vi "Feed Module Tags.vi"(0 "Feed Module Configs":T1[](array[typedef]) {"Settings"."Bronkhorst M14 Settings"."Smoothing Steps" min=1 step=1; "Settings"."Ismatech 3 Channel Settings"."Channel Number" min=0 max=3; "Settings"."Ismatech 3 Channel Settings"."Pump Number" min=1; "Settings"."PID range"."PID Low" min=0.0 max=100.0 format="%.2f"; "Settings"."PID range"."PID High" format="%.2f"; "Settings"."PID 2 Parameters"."PID gains"."derivative time (Td, min)" format="%.3f"; "Settings"."PID 2 Parameters"."PID gains"."integral time (Ti, min)" format="%.3f"; "Settings"."PID 2 Parameters"."PID gains"."proportional gain (Kc)" format="%.3f"; "Settings"."Bronkhorst M13 Flow Meter"."Smoothing Steps" min=1 step=1; "Settings"."ASIA Pump C"."channel" min=0 max=1 step=1; "Settings"."Ismatech"."Pump Number" min=1.0 max=20.0 step=1.0; "Settings"."Masterflex"."Pump Number" min=1.0 max=20.0 step=1.0}) -> (2 "All  Flow Meter Tags":string[](array[string]), 3 "All  Scale Tags":string[](array[string]), 4 "All  Numeric Tags":string[](array[string]), 6 "Pump Flow Tag":string, 8 "Feed Module Tag Names":T22, 10 "Feed Module Tags Array":T22[](array[typedef]), 12 "Scale Tag":string, 13 "All Boolean Tags":string[](array[string]), 14 "PID 2 Out Tag":string)   [LabVIEW 2018]
uses:
  Feed Module/Controls/Feed Module Tag Names Cluster.ctl
  Feed Module/Controls/Feed Module Config Cluster.ctl
  <vilib>/Utility/miscctls.llb/LVPoint32TypeDef.ctl
  Feed Module/Controls/Feed Module Settings Cluster.ctl
  Ismatec ISM 831C/Controls/Ismatech ISM831C Settings Cluster.ctl
  Masterflex 7550-30/Controls/Settings Cluster.ctl
  Mettler Toledo/Controls/Settings Cluster.ctl
  Bronkhorst M13 Flow Meter/Settings Cluster.ctl
  Measure Instrument/PID 2 Parameters Cluster.ctl
  Measure Instrument/PID Input Enum.ctl
  Measure Instrument/PID 2 Output Enum.ctl
  Tacmina QI/Tacmina QI DAQ Setting.ctl
  KNF Pump/Settings Cluster plus SIMDOS.ctl
  ASIA Pump/Pump Settings.ctl
  VICI M50 Party Mode/Settings Cluster.ctl
  FLOM Pump/Settings Cluster.ctl
  SSI PR Class/SSI PR or LD Settings Cluster.ctl
  Masterflex 75211/Masterflex 75211 DAQ Setting.ctl
  SSI PR Class/SSI P40 Settings Cluster.ctl
  Ismatec 78001/Ismatec 4083.ctl
  Bronkhorst M14 Flow Meter/Settings Cluster.ctl
  Tag VIs/Numeric Alarm Settings Cluster.ctl
  Feed Module/Feed Module.lvlib
  Masterflex 7550-30/Masterflex 7550-30.lvlib
  Ismatec ISM 831C/Ismatec ISM 831C.lvlib
  Tacmina QI/Tacmina QI.lvlib
  KNF Pump/KNF SIMDOS.lvlib
  VICI M50 Party Mode/VICI M6 M50 Party Mode.lvlib
  FLOM Pump/FLOM Pump.lvlib
  ASIA Pump.lvlib
  Mettler Toledo/Mettler Toledo.lvlib
  Bronkhorst M13 Flow Meter/Bronkhorst M13 Flow Meter.lvlib
  SSI PR Class/SSI PR or LD Pump.lvlib
  Masterflex 75211/Masterflex 75211.lvlib
  SSI PR Class/SSI P40 Pump.lvlib
  Ismatec 78001/Ismatec 4308.lvlib
  Bronkhorst M14 Flow Meter/Bronkhorst M14 Flow Meter.lvlib
panel:
  # "Output Instruments"
  # "Input Instruments"
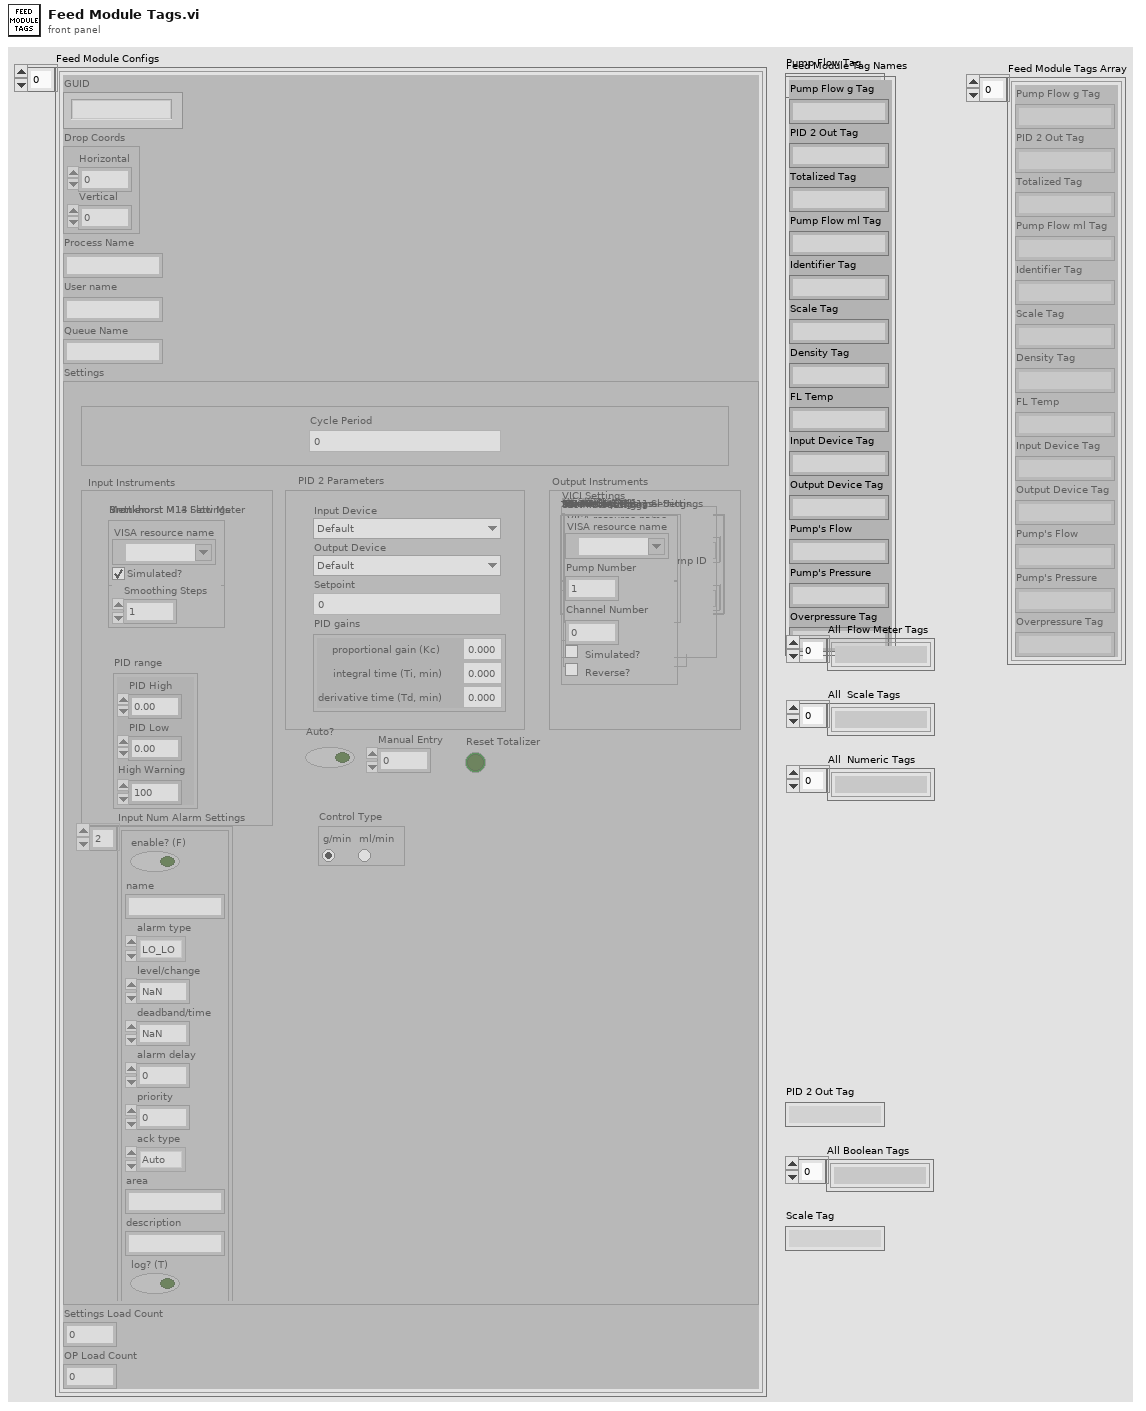
[diagram p1: front panel]
types:
  T1 = typedef "Feed Module.lvlib/Feed Module Config Cluster.ctl" = cluster{"GUID":string, "Drop Coords":T2, "Process Name":string, "User name":string, "Queue Name":string, "Settings":T3, "Settings Load Count":i32, "OP Load Count":i32}
  T2 = typedef "LVPoint32TypeDef.ctl" = cluster{"Horizontal":i32, "Vertical":i32}
  T3 = typedef "Feed Module.lvlib/Feed Module Settings Cluster.ctl" = cluster{"Cycle Period":dbl, "Ismatech":T4, "Masterflex":T5, "Mettler":T6, "Bronkhorst M13 Flow Meter":T7, "PID 2 Parameters":T8, "Manual Entry":dbl, "Auto?":bool, "PID range":cluster{"PID High":dbl, "PID Low":dbl, "High Warning":dbl}, "Tacmina Settings":T11, "KNF SIMDOS Settings":T12, "ASIA Pump C":T13, "VICI Settings":T14, "FLOM Settings":T15, "SSI PR/LD Settings":T16, "Masterflex 75211 Settings":T17, "SSI P40 Settings":T18, "Ismatech 3 Channel Settings":T19, "Bronkhorst M14 Settings":T20, "Reset Totalizer":bool, "Input Num Alarm Settings":T21[], "Control Type":enum32{"g/min", "ml/min"}}
  T4 = typedef "Ismatec ISM 831C.lvlib/Ismatech ISM831C Settings Cluster.ctl" = cluster{"VISA resource name":refnum<visa-resource-name>, "Simulated?":bool, "Pump Number":dbl, "Reverse?":bool}
  T5 = typedef "Masterflex 7550-30.lvlib/Settings Cluster.ctl" = cluster{"VISA resource name":refnum<visa-resource-name>, "Simulated?":bool, "Pump Number":dbl, "Reverse?":bool}
  T6 = typedef "Mettler Toledo.lvlib/Settings Cluster.ctl" = cluster{"VISA resource name":refnum<visa-resource-name>, "Simulated?":bool}
  T7 = typedef "Bronkhorst M13 Flow Meter.lvlib/Settings Cluster.ctl" = cluster{"VISA resource name":refnum<visa-resource-name>, "Simulated?":bool, "Smoothing Steps":i32}
  T8 = typedef "PID 2 Parameters Cluster.ctl" = cluster{"Input Device":T9, "Output Device":T10, "Setpoint":dbl, "PID gains":cluster{"proportional gain (Kc)":dbl, "integral time (Ti, min)":dbl, "derivative time (Td, min)":dbl}}
  T9 = typedef "PID Input Enum.ctl" = enum16{"Default", "Bronkhorst M13", "Bronkhorst M14", "Scale Rate of Change"}
  T10 = typedef "PID 2 Output Enum.ctl" = enum16{"Default", "Ismatec ISM 4308", "Ismatec ISM 831C", "Masterflex 7550-30", "VICI M6", "VICI M50", "Tacmina QI", "KNF SIMDOS", "ASIA Type C", "FLOM UI-22-11", "SSI PR/LD", "SSI P40", "Masterflex 75211-70"}
  T11 = typedef "Tacmina QI.lvlib/Tacmina QI DAQ Setting.ctl" = cluster{"Analog DAQ Task":refnum<k21>, "Digital DAQ Task":refnum<k21>}
  T12 = typedef "KNF SIMDOS.lvlib/Settings Cluster plus SIMDOS.ctl" = cluster{"VISA resource name":refnum<visa-resource-name>, "Simulated?":bool}
  T13 = typedef "ASIA Pump.lvlib/Pump Settings.ctl" = cluster{"ASIA Pump #":i32, "channel":i32, "Simulated":bool}
  T14 = typedef "VICI M6 M50 Party Mode.lvlib/Settings Cluster.ctl" = cluster{"VISA resource name":refnum<visa-resource-name>, "Pump ID":string, "Pump Head Vol":dbl, "Reverse?":bool, "Simulated?":bool}
  T15 = typedef "FLOM Pump.lvlib/Settings Cluster.ctl" = cluster{"VISA resource name":refnum<visa-resource-name>, "Simulated?":bool, "Pump Number":dbl}
  T16 = typedef "SSI PR or LD Pump.lvlib/SSI PR or LD Settings Cluster.ctl" = cluster{"VISA resource name":refnum<visa-resource-name>, "Simulated?":bool}
  T17 = typedef "Masterflex 75211.lvlib/Masterflex 75211 DAQ Setting.ctl" = cluster{"Analog DAQ Task":refnum<k21>, "Digital DAQ Task":refnum<k21>}
  T18 = typedef "SSI P40 Pump.lvlib/SSI P40 Settings Cluster.ctl" = cluster{"VISA resource name":refnum<visa-resource-name>, "Simulated?":bool}
  T19 = typedef "Ismatec 4308.lvlib/Ismatec 4083.ctl" = cluster{"VISA resource name":refnum<visa-resource-name>, "Pump Number":i16, "Channel Number":i16, "Simulated?":bool, "Reverse?":bool}
  T20 = typedef "Bronkhorst M14 Flow Meter.lvlib/Settings Cluster.ctl" = cluster{"VISA resource name":refnum<visa-resource-name>, "Simulated?":bool, "Smoothing Steps":i32}
  T21 = typedef "Numeric Alarm Settings Cluster.ctl" = cluster{"enable? (F)":bool, "name":string, "alarm type":enum16{"HI_HI", "HI", "LO", "LO_LO"}, "level/change":dbl, "deadband/time":dbl, "alarm delay":dbl, "priority":u32, "ack type":enum16{"Auto", "User", "None", "Each Occurrence"}, "area":string, "description":string, "log? (T)":bool}
  T22 = typedef "Feed Module.lvlib/Feed Module Tag Names Cluster.ctl" = cluster{"Pump Flow g Tag":string, "PID 2 Out Tag":string, "Totalized Tag":string, "Pump Flow ml Tag":string, "Identifier Tag":string, "Scale Tag":string, "Density Tag":string, "FL Temp":string, "Input Device Tag":string, "Output Device Tag":string, "Pump's Flow":string, "Pump's Pressure":string, "Overpressure Tag":string}
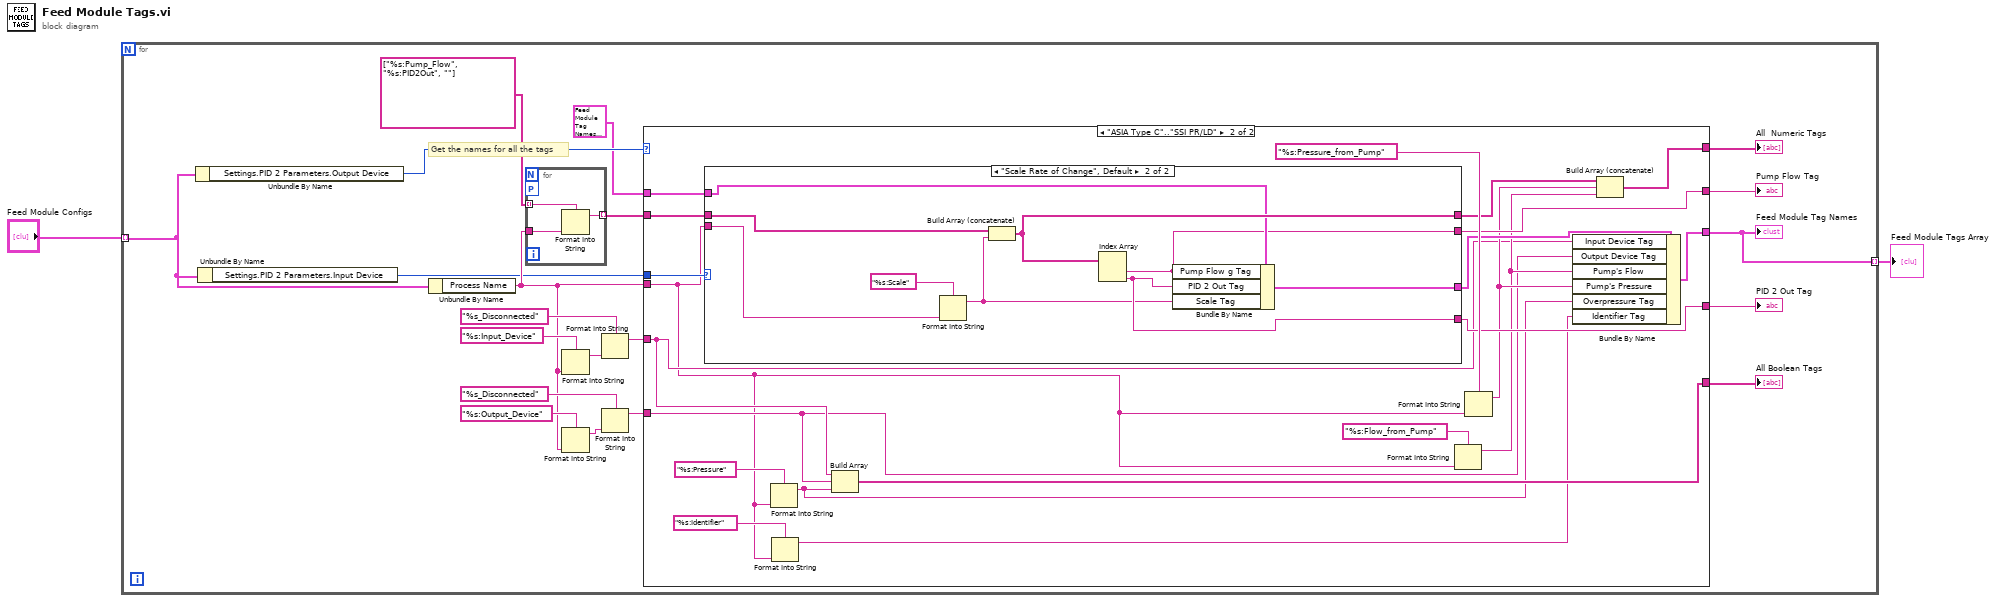
[diagram p0: block diagram]
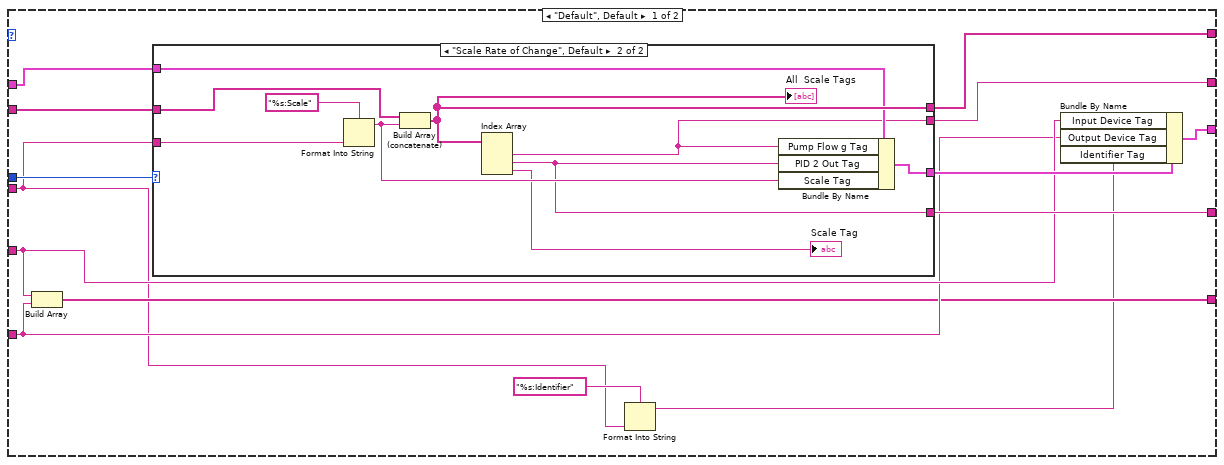
[diagram p2: hidden frame]
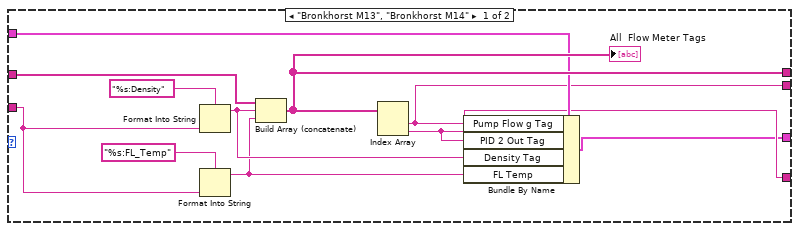
[diagram p3: hidden frame]
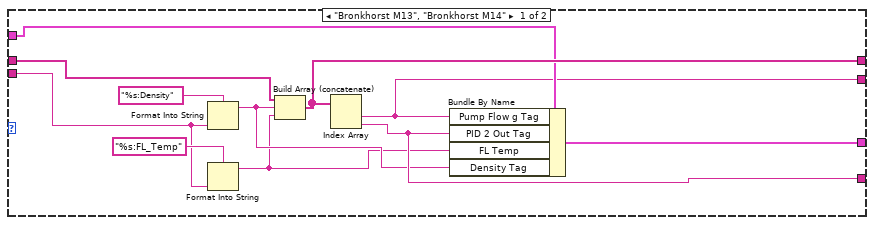
[diagram p4: hidden frame]
diagram:
  n1 = for {
    tunnel: "Feed Module Configs" -> [w5] mode=indexing
    tunnel: [w4] -> w2 mode=indexing
    # "Get the names for all the tags"
    n2 = Unbundle By Name(w5) -> ("Settings.PID 2 Parameters.Output Device"=w15:T10)
    n3 = Unbundle By Name(w5) -> ("Settings.PID 2 Parameters.Input Device"=w13:T9)
    n4 = Unbundle By Name(w5) -> ("Process Name"=w14:string)
    n5 = for {
      tunnel: string[] ["%s:Pump_Flow", "%s:PID2Out", ""] -> [w101] mode=indexing
      tunnel: w14 -> [w100]
      tunnel: [w99] -> w12 mode=indexing
      workers-P: _ -> [_]
      n6 = Format Into String(format string=w101, w100) -> (resulting string=w99:string)  [unwired: 2 in, 1 out]
    }
    n7 = Format Into String(format string="%s:Input_Device", w14) -> (resulting string=w19:string)  [unwired: 2 in, 1 out]
    n8 = Format Into String(format string="%s:Output_Device", w14) -> (resulting string=w18:string)  [unwired: 2 in, 1 out]
    n9 = Format Into String(format string="%s_Disconnected", w19) -> (resulting string=w8:string)  [unwired: 2 in, 1 out]
    n10 = Format Into String(format string="%s_Disconnected", w18) -> (resulting string=w7:string)  [unwired: 2 in, 1 out]
    n11 = case shown="\"ASIA Type C\"..\"SSI PR/LD\"" w15 {
      tunnel: w14 -> [w23 w59]
      tunnel: w13 -> [w36 w76]
      tunnel: w12 -> [w35 w75]
      tunnel: [w34 w74] -> w11
      tunnel: [w33 w72] -> w9
      tunnel: [w32 w71] -> w10
      tunnel: [w31 w69] -> w4
      tunnel: w8 -> [w29 w65]
      tunnel: w7 -> [w28 w64]
      tunnel: [w27 w63] -> w6
      tunnel: T22 {"Pump Flow g Tag"="", "PID 2 Out Tag"="", "Totalized Tag"="", "Pump Flow ml Tag"="", "Identifier Tag"="", "Scale Tag"="", "Density Tag"="", "FL Temp"="", "Input Device Tag"="", "Output Device Tag"="", "Pump's Flow"="", "Pump's Pressure"="", "Overpressure Tag"=""} ("Feed Module Tag Names") -> [w26 w61]
      frame "Default", Default {
        n12 = Build Array(w29, w28) -> (w27:string[])
        n13 = case shown="\"Scale Rate of Change\", Default" w36 {
          tunnel: w35 -> [w45 w57]
          tunnel: [w43 w54] -> w34
          tunnel: w23 -> [w44 w55]
          tunnel: [w41 w51] -> w32
          tunnel: [w40 w49] -> w33
          tunnel: w26 -> [w42 w53]
          tunnel: [w39 w52] -> w30
          frame "Bronkhorst M13", "Bronkhorst M14" {
            n14 = Format Into String(format string="%s:Density", w44) -> (resulting string=w38:string)  [unwired: 2 in, 1 out]
            n15 = Format Into String(format string="%s:FL_Temp", w44) -> (resulting string=w37:string)  [unwired: 2 in, 1 out]
            n16 = Build Array (concatenate)(w45, w38, w37) -> (w43:string[])
            "All  Flow Meter Tags" <- w43
            n17 = Index Array(array=w43) -> (element #1=w41:string, element #2=w40:string)  [unwired: 2 in]
            n18 = Bundle By Name(cluster=w42, "Pump Flow g Tag"=w41, "PID 2 Out Tag"=w40, "Density Tag"=w38, "FL Temp"=w37) -> (w39:T22)
          }
          frame "Scale Rate of Change", Default {
            n19 = Format Into String(format string="%s:Scale", w55) -> (resulting string=w50:string)  [unwired: 2 in, 1 out]
            n20 = Build Array (concatenate)(w57, w50) -> (w54:string[])
            "All  Scale Tags" <- w54
            n21 = Index Array(array=w54) -> (element #1=w51:string, element #2=w49:string, element #3=→"Scale Tag":string)  [unwired: 3 in]
            n22 = Bundle By Name(cluster=w53, "Pump Flow g Tag"=w51, "PID 2 Out Tag"=w49, "Scale Tag"=w50) -> (w52:T22)
          }
        }
        n23 = Format Into String(format string="%s:Identifier", w23) -> (resulting string=w24:string)  [unwired: 2 in, 1 out]
        n24 = Bundle By Name(cluster=w30, "Input Device Tag"=w29, "Output Device Tag"=w28, "Identifier Tag"=w24) -> (w31:T22)
      }
      frame "ASIA Type C".."SSI PR/LD" {
        n25 = case shown="\"Scale Rate of Change\", Default" w76 {
          tunnel: w75 -> [w87 w98]
          tunnel: [w85 w95] -> w73
          tunnel: w59 -> [w86 w96]
          tunnel: [w83 w91] -> w71
          tunnel: [w82 w92] -> w72
          tunnel: w61 -> [w84 w94]
          tunnel: [w81 w93] -> w70
          frame "Bronkhorst M13", "Bronkhorst M14" {
            n26 = Format Into String(format string="%s:Density", w86) -> (resulting string=w80:string)  [unwired: 2 in, 1 out]
            n27 = Format Into String(format string="%s:FL_Temp", w86) -> (resulting string=w79:string)  [unwired: 2 in, 1 out]
            n28 = Build Array (concatenate)(w87, w80, w79) -> (w85:string[])
            n29 = Index Array(array=w85) -> (element #1=w83:string, element #2=w82:string)  [unwired: 2 in]
            n30 = Bundle By Name(cluster=w84, "Pump Flow g Tag"=w83, "PID 2 Out Tag"=w82, "FL Temp"=w79, "Density Tag"=w80) -> (w81:T22)
          }
          frame "Scale Rate of Change", Default {
            n31 = Format Into String(format string="%s:Scale", w96) -> (resulting string=w90:string)  [unwired: 2 in, 1 out]
            n32 = Build Array (concatenate)(w98, w90) -> (w95:string[])
            n33 = Index Array(array=w95) -> (element #1=w91:string, element #2=w92:string)  [unwired: 2 in]
            n34 = Bundle By Name(cluster=w94, "Pump Flow g Tag"=w91, "PID 2 Out Tag"=w92, "Scale Tag"=w90) -> (w93:T22)
          }
        }
        n35 = Format Into String(format string="%s:Pressure", w59) -> (resulting string=w62:string)  [unwired: 2 in, 1 out]
        n36 = Format Into String(format string="%s:Identifier", w59) -> (resulting string=w58:string)  [unwired: 2 in, 1 out]
        n37 = Build Array(w65, w64, w62) -> (w63:string[])
        n38 = Format Into String(format string="%s:Flow_from_Pump", w59) -> (resulting string=w67:string)  [unwired: 2 in, 1 out]
        n39 = Format Into String(format string="%s:Pressure_from_Pump", w59) -> (resulting string=w68:string)  [unwired: 2 in, 1 out]
        n40 = Bundle By Name(cluster=w70, "Input Device Tag"=w65, "Output Device Tag"=w64, "Pump's Flow"=w67, "Pump's Pressure"=w68, "Overpressure Tag"=w62, "Identifier Tag"=w58) -> (w69:T22)
        n41 = Build Array (concatenate)(w73, w68, w67) -> (w74:string[])
      }
    }
    "All  Numeric Tags" <- w11
    "All Boolean Tags" <- w6
    "PID 2 Out Tag" <- w9
    "Pump Flow Tag" <- w10
    "Feed Module Tag Names" <- w4
  }
  "Feed Module Tags Array" <- w2
